vi "Stop Core.vi"(10 "final error code":i32, 11 "UI Actor in":refnum<class "UI Actor.lvclass">) -> (3 "UI Actor out":refnum<class "UI Actor.lvclass">)   [LabVIEW 2013, in "SET Project Editor.lvlib" / "UI Actor.lvclass"]
doc: "(<B>Filename</B>: Actor Framework.lvlib:Actor.lvclass:Stop Core.vi)\n\nDefines what the actor does before it stops. Use the <B>final error code</B> input to determine whether the actor shut down in response to an error.\n\nBy default, this method does nothing. A descendant class may override it to define behavior, such as shutting down any processes the actor initiated in its override of the Actor Core method."
uses:
  UI Actor.lvclass
  <vilib>/ActorFramework/Actor/Actor.lvclass
  UI Actor.lvclass/UI Actor.ctl
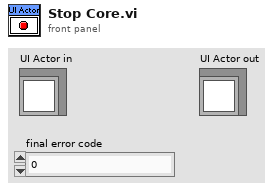
[diagram p1: front panel]
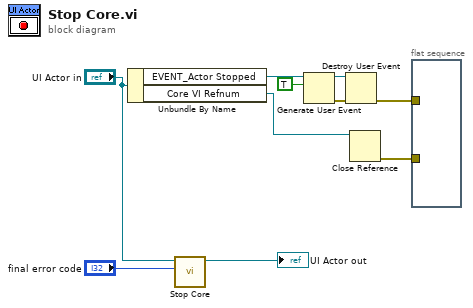
[diagram p0: block diagram]
diagram:
  n1 = Unbundle By Name("UI Actor in") -> ("EVENT_Actor Stopped"=w5:refnum<user-event>, "Core VI Refnum"=w2:refnum<vi>)
  n2 = call-parent "Stop Core.vi"("final error code"="final error code", "Actor in"="UI Actor in") -> ("Actor out"=→"UI Actor out":refnum<class "UI Actor.lvclass">)  [unwired: 9 in]
  n3 = Generate User Event(user event=w5, event data cluster=TRUE ("event data")) -> (user event out=w7:refnum<user-event>, error out=w8:errorcluster)  [unwired: 2 in]
  n4 = Destroy User Event(user event=w7, error in=w8) -> (error out=w3:errorcluster)
  n5 = Close Reference(reference=w2) -> (error out=w1:errorcluster)  [unwired: 1 in]
  n6 = flat-sequence {
    tunnel: w3 -> [_]
    tunnel: w1 -> [_]
    frame #0 {
    }
  }
